vi "XY Graph Add Plot to Sum.vi"(6 "epsilon (machine)":dbl=2.220446049250313e-16, 7 "Keep Plot":bool, 8 "Sum Plot Y":dbl[](array[numeric]), 9 "Sum Plot X":dbl[](array[numeric]), 10 "New Plot Y":dbl[](array[numeric]), 11 "New Plot X":dbl[](array[numeric])) -> (0 "Sum Plot Y":dbl[](array[numeric]))   [LabVIEW 2021, in "XY Graph Add-Ons.lvlib"]
uses:
  XY Graph Add-Ons.lvlib
  Arrays/Arrays.lvlib
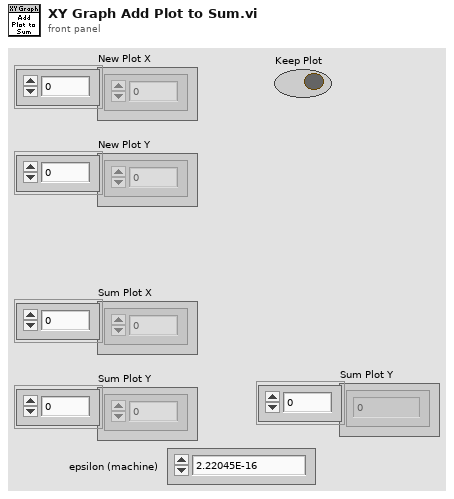
[diagram p1: front panel]
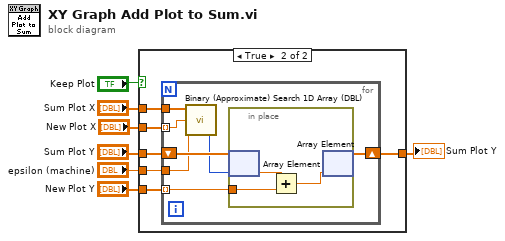
[diagram p0: block diagram]
diagram:
  n1 = case shown="True" "Keep Plot" {
    tunnel: [w8 w10] -> w5
    tunnel: "Sum Plot Y" -> [w8 w12]
    tunnel: "Sum Plot X" -> [_ w14]
    tunnel: "New Plot X" -> [_ w13]
    tunnel: "New Plot Y" -> [_ w11]
    tunnel: "epsilon (machine)" -> [_ w9]
    frame False {
    }
    frame True {
      n2 = for {
        tunnel: w14 -> [w21]
        tunnel: w13 -> [w20] mode=indexing
        shift-right: [w18] -> w10
        shift-left: w12 -> [w19]
        tunnel: w11 -> [w16] mode=indexing
        tunnel: w9 -> [w15]
        n3 = call "Binary (Approximate) Search 1D Array (DBL).vi"("epsilon (machine)"=w15, "element"=w20, "1D array"=w21) -> ("index"=w17:i32)
        n4 = in-place {
          in-place-border: w16 -> [w23]
          n5 = in-place-array #1(w19, w17) -> (w24:dbl)
          n6 = Add(x=w24, y=w23) -> (x+y=w22:dbl)
          n7 = in-place-array #1(w22) -> (w18:dbl[])  [unwired: 1 out]
        }
      }
    }
  }
  "Sum Plot Y" <- w5
